vi "average1.vi"(6 "Size":i32=100, 7 "SignalIn":waveform(dbl)) -> (3 "output waveform":waveform(dbl))   [LabVIEW 2010]
doc: "Acquires a large number of data points and compresses the data points into a smaller number of points.\n--------------------\n\nThis Express VI is configured as follows:\n\nReduction Factor: 100\nReduction Method: Mean"
panel:
  out "LastIndex":i32
  # "Усреднение с сохранением фазы"
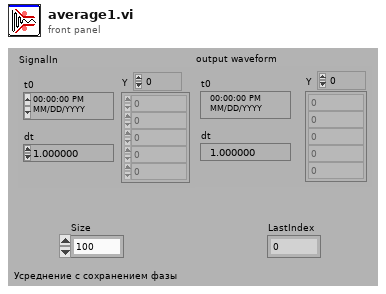
[diagram p1: front panel]
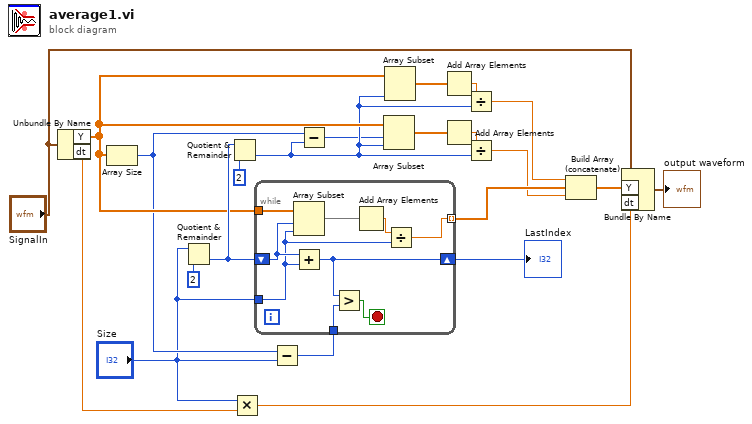
[diagram p0: block diagram]
diagram:
  n1 = Unbundle By Name("SignalIn") -> ("Y"=w13:dbl[], "dt"=w5:dbl)
  n2 = Array Size(array=w13) -> (size(s)=w9:i32)
  n3 = Quotient & Remainder(x="Size", y=2) -> (floor(x/y)=w15:i32)  [unwired: 1 out]
  n4 = Quotient & Remainder(x=w15, y=2) -> (floor(x/y)=w8:i32)  [unwired: 1 out]
  n5 = Multiply(x="Size", y=w5) -> (x*y=w21:dbl)
  n6 = Subtract(x=w9, y="Size") -> (x-y=w16:i32)
  n7 = while {
    tunnel: w13 -> [w31]
    tunnel: [w23] -> w19 mode=indexing
    tunnel: "Size" -> [w25]
    shift-right: [w29] -> w20
    shift-left: w15 -> [w30]
    tunnel: w16 -> [w28]
    stop <- w27 stop-if-true
    n8 = Array Subset(array=w31, index=w30, length=w25) -> (w24:dbl[])
    n9 = Add(x=w30, y=w25) -> (x+y=w29:i32)
    n10 = Greater?(x=w29, y=w28) -> (0:w27:bool)
    n11 = Add Array Elements(numeric array=w24) -> (sum=w26:dbl)
    n12 = Divide(x=w26, y=w25) -> (x/y=w23:dbl)
  }
  "LastIndex" <- w20
  n13 = Subtract(x=w9, y=w8) -> (x-y=w7:i32)
  n14 = Array Subset(array=w13, index=w7, length=w8) -> (w2:dbl[])
  n15 = Array Subset(array=w13, length=w8) -> (w1:dbl[])  [unwired: 1 in]
  n16 = Add Array Elements(numeric array=w1) -> (sum=w12:dbl)
  n17 = Add Array Elements(numeric array=w2) -> (sum=w11:dbl)
  n18 = Divide(x=w12, y=w8) -> (x/y=w3:dbl)
  n19 = Divide(x=w11, y=w8) -> (x/y=w4:dbl)
  n20 = Build Array (concatenate)(w3, w19, w4) -> (w10:dbl[])
  n21 = Bundle By Name(cluster="SignalIn", "Y"=w10, "dt"=w21) -> (→"output waveform":waveform(dbl))
